vi "gradient_ascent_test_2d_v2.vi"() -> ()   [LabVIEW 2024]
uses:
  <vilib>/Math Plots/3D Math Plots/3D Scatter/3D Scatter XCtrl/3D Scatter.xctl
  <vilib>/Math Plots/3D Math Plots/3D Scatter/3D Scatter Datatype/Public/Plot Helper (Vector).vi
  <vilib>/Math Plots/3D Math Plots/3D Scatter/3D Scatter Datatype/3D Scatter Datatype.lvclass
panel:
  out "3D Scatter":refnum<class "3D Plot Datatype.lvclass">[](xcontrol)
  out "Intensity Graph":dbl[][](graph)
  in  "N trials":dbl=16.0
  out "diff":dbl[](array[numeric])
  out "end result":dbl[](array[numeric])
  in  "k":dbl=150.0
  out "StdDev":dbl[](array[numeric])
  out "Mean":dbl[](array[numeric])
  # "Used only to create Gaussian to optimize"
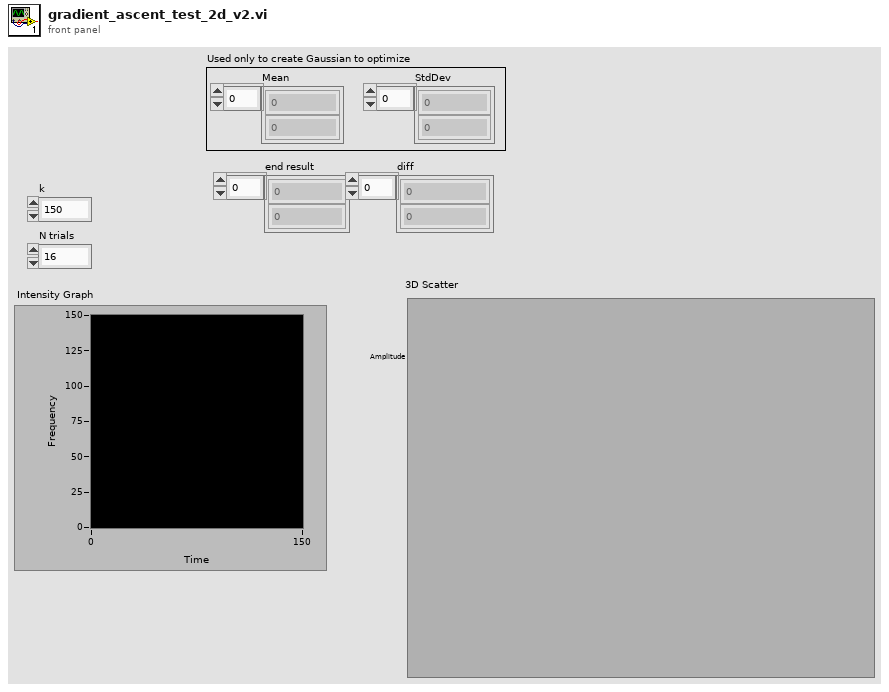
[diagram p1: front panel]
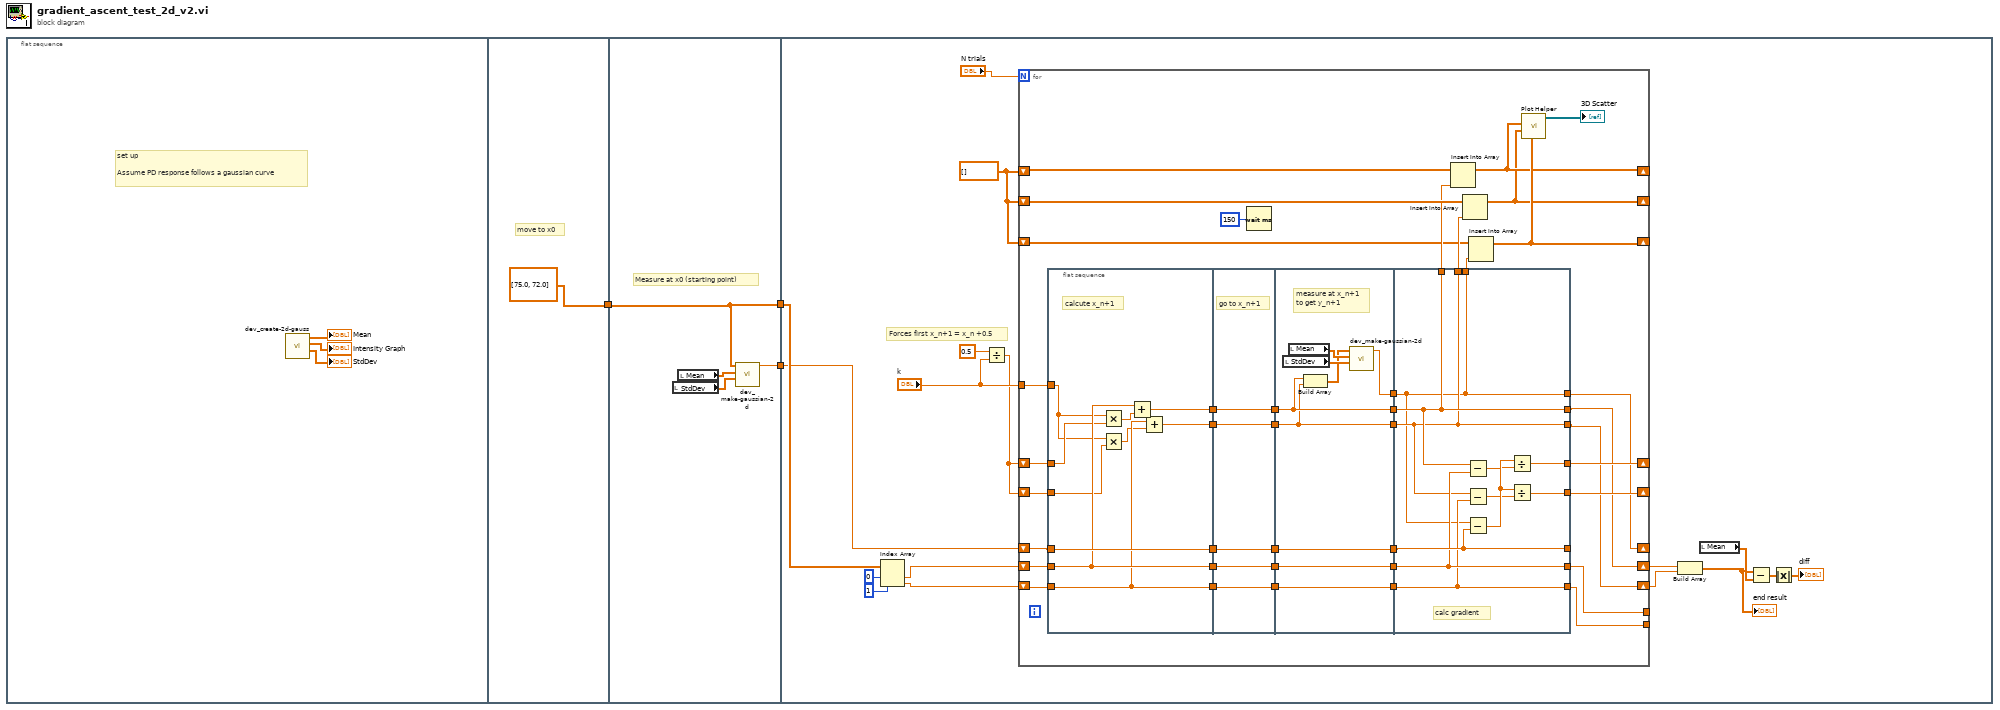
[diagram p0: block diagram]
diagram:
  n1 = flat-sequence {
    tunnel: [dbl[] [75.0, 72.0]] -> w1
    tunnel: [w8] -> w3
    tunnel: [w9] -> w2
    tunnel: w1 -> [w9]
    tunnel: w3 -> [w27]
    tunnel: w2 -> [w28]
    frame #0 {
      # "set up\n\nAssume PD response follows a gaussian curve"
      n2 = call "dev_create-2d-gauss.vi"() -> ("StdDev"=→"StdDev":dbl[], "Intensity Graph"=→"Intensity Graph":dbl[][], "Mean"=→"Mean":dbl[])  [unwired: 9 in]
    }
    frame #1 {
      # "move to x0"
    }
    frame #2 {
      # "Measure at x0 (starting point)"
      n3 = local read "StdDev"() -> (w10:dbl[])
      n4 = local read "Mean"() -> (w11:dbl[])
      n5 = call "dev_make-gaussian-2d.vi"("StdDev"=w10, "Mean"=w11, "in"=w9) -> ("out"=w8:dbl)  [unwired: 8 in]
    }
    frame #3 {
      w15 = dbl[] []
      # "Forces first x_n+1 = x_n +0.5"
      n6 = Index Array(array=w28, index #1=0 ("index"), index #2=1 ("index")) -> (element #1=w18:dbl, element #2=w17:dbl)
      n7 = Divide(x=0.5, y="k") -> (x/y=w16:dbl)
      n8 = for {
        N: "N trials" -> [_]
        shift-right: [w39] -> w13
        shift-left: w18 -> [w57]
        shift-right: [w40] -> _
        shift-left: w27 -> [w58]
        tunnel: "k" -> [w68]
        shift-right: [w32] -> _
        shift-left: w15 -> [w60]
        shift-right: [w31] -> _
        shift-left: w15 -> [w59]
        shift-right: [w38] -> w12
        shift-left: w17 -> [w50]
        shift-right: [w43] -> _
        shift-left: w16 -> [w41]
        shift-right: [w44] -> _
        shift-left: w16 -> [w42]
        shift-right: [w33] -> _
        shift-left: w15 -> [w35]
        tunnel: [w30] -> _
        tunnel: [w29] -> _
        n9 = flat-sequence {
          tunnel: w68 -> [w69]
          tunnel: [w78] -> w67
          tunnel: w58 -> [w77]
          tunnel: [w77] -> w64
          tunnel: w57 -> [w76]
          tunnel: [w76] -> w55
          tunnel: [w75] -> w51
          tunnel: w50 -> [w75]
          tunnel: [w73] -> w48
          tunnel: w42 -> [w72]
          tunnel: w41 -> [w70]
          tunnel: w67 -> [w83]
          tunnel: [w83] -> w66
          tunnel: w64 -> [w82]
          tunnel: [w82] -> w63
          tunnel: [w81] -> w56
          tunnel: w55 -> [w81]
          tunnel: [w80] -> w52
          tunnel: w51 -> [w80]
          tunnel: w48 -> [w79]
          tunnel: [w79] -> w47
          tunnel: w66 -> [w86]
          tunnel: [w86] -> w65
          tunnel: w63 -> [w92]
          tunnel: [w92] -> w62
          tunnel: w56 -> [w91]
          tunnel: [w91] -> w54
          tunnel: w52 -> [w90]
          tunnel: [w90] -> w49
          tunnel: w47 -> [w85]
          tunnel: [w85] -> w46
          tunnel: [w84] -> w45
          tunnel: w65 -> [w98]
          tunnel: w62 -> [w103]
          tunnel: w54 -> [w102]
          tunnel: [w97] -> w37
          tunnel: [w98] -> w53
          tunnel: w49 -> [w101]
          tunnel: [w98] -> w39
          tunnel: w46 -> [w97]
          tunnel: [w97] -> w38
          tunnel: w45 -> [w93]
          tunnel: [w93] -> w40
          tunnel: [w103] -> _
          tunnel: [w102] -> w30
          tunnel: [w101] -> w29
          tunnel: [w100] -> w44
          tunnel: [w99] -> w43
          tunnel: [w93] -> w36
          frame #0 {
            # "calcute x_n+1"
            n10 = Multiply(x=w69, y=w72) -> (x*y=w74:dbl)
            n11 = Multiply(x=w69, y=w70) -> (x*y=w71:dbl)
            n12 = Add(x=w76, y=w74) -> (x+y=w78:dbl)
            n13 = Add(x=w75, y=w71) -> (x+y=w73:dbl)
          }
          frame #1 {
            # "go to x_n+1"
          }
          frame #2 {
            # "measure at x_n+1\nto get y_n+1"
            n14 = local read "StdDev"() -> (w88:dbl[])
            n15 = local read "Mean"() -> (w89:dbl[])
            n16 = Build Array(w86, w85) -> (w87:dbl[])
            n17 = call "dev_make-gaussian-2d.vi"("StdDev"=w88, "Mean"=w89, "in"=w87) -> ("out"=w84:dbl)  [unwired: 8 in]
          }
          frame #3 {
            # "calc gradient"
            n18 = Subtract(x=w98, y=w102) -> (x-y=w94:dbl)
            n19 = Subtract(x=w97, y=w101) -> (x-y=w95:dbl)
            n20 = Subtract(x=w93, y=w103) -> (x-y=w96:dbl)
            n21 = Divide(x=w96, y=w94) -> (x/y=w100:dbl)
            n22 = Divide(x=w96, y=w95) -> (x/y=w99:dbl)
          }
        }
        n23 = Wait (ms)(milliseconds to wait=u32 150) -> ()  [unwired: 1 out]
        n24 = Insert Into Array(array=w60, new element=w53) -> (w32:dbl[])  [unwired: 1 in]
        n25 = Insert Into Array(array=w59, new element=w37) -> (w31:dbl[])  [unwired: 1 in]
        n26 = Insert Into Array(array=w35, new element=w36) -> (w33:dbl[])  [unwired: 1 in]
        n27 = call-poly <vilib>:"Plot Helper.vi"("z vector"=w33, "y vector"=w31, "x vector"=w32) -> ("3D Plot lvclass Array out"=→"3D Scatter":refnum<class "3D Plot Datatype.lvclass">[])  [unwired: 3 in, 5 out]
      }
      n28 = Build Array(w13, w12) -> (w14:dbl[])
      "end result" <- w14
      n29 = local read "Mean"() -> (w26:dbl[])
      n30 = Subtract(x=w14, y=w26) -> (x-y=w25:dbl[])
      n31 = Absolute Value(x=w25) -> (abs(x)=→"diff":dbl[])
    }
  }
